vi "6812B_AC.vi"() -> ()   [LabVIEW 2019]
doc: "Shows how to generate a standard output."
uses:
  <instrlib>/Agilent 681x Series/Agilent 681x Series.lvlib
panel:
  out "PwrMeas":T1
  out "CurMeas":T2
  out "CUR":T3(graph)={"Peak Current"=0.0194168, "AC RMS Current"=0.00868389, "AC + DC RMS Current"=0.00868755}
  out "POT":T4(graph)={"Reactive Power"=0.130219, "Real Power"=0.000577786, "Apparent Power"=0.13022}
  in  "STOP":bool
  in  "Pulse Characteristic Value (%)":dbl=100.0 format="%#.4g"
  in  "Pulse Characteristic (0: Duty Cycle)":u16(ring) items=["Duty Cycle", "Pulse Width"]
  in  "Period (s)":dbl=10.0 format="%#.4g"
  in  "Trigger Delay (s)":dbl=10.0 format="%#.5g"
  in  "Pulse Count":dbl=1.0 format="%#.4g"
  in  "Voltage Mode (0: Fix)":u16(ring) items=["Fixed", "Step", "Pulse", "List"]
  in  "Triggered Voltage Amplitude (V)":dbl=1.0 format="%#.4g"
  in  "Peak Current Limit (13 A)":dbl=13.0 format="%#.4g"
  in  "RMS Current Limit (1 A)":dbl=1.0 format="%#.4g"
  in  "Voltage Amplitude (1.0 V)":dbl=1.0 format="%#.4g"
  in  "Output Frequency (60 Hz)":dbl=60.0 format="%#.4g"
  in  "Output Waveform Type (0: Sinusoid)":u16(ring) items=["Sinusoid", "Square", "Clipped Sinusoid", "User Specified"]
  in  "VISA resource name":refnum<visa-resource-name>
  # "(c) 2008-2021 National Instruments Corp.  ALL RIGHTS RESERVED."
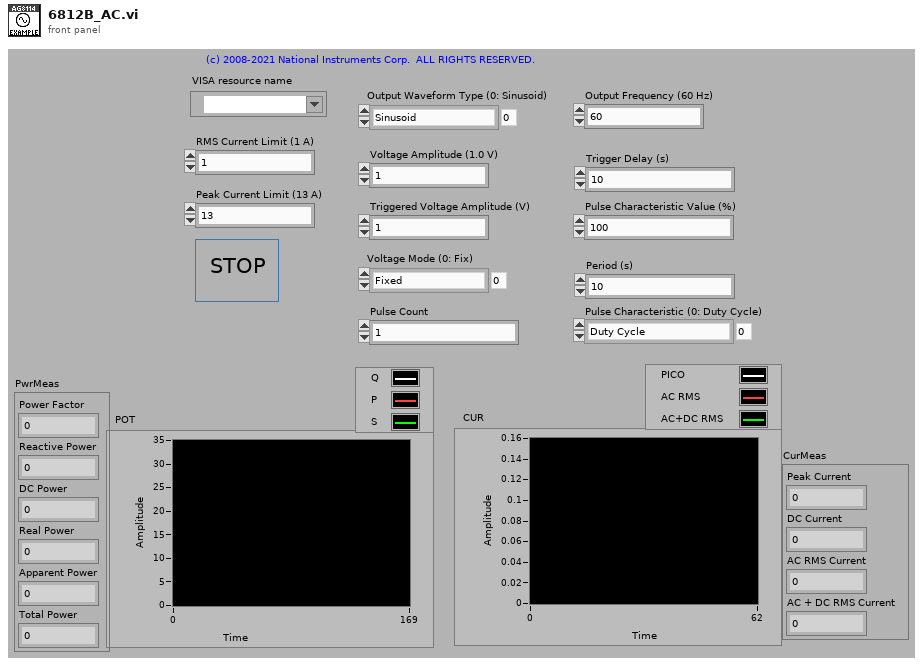
[diagram p1: front panel]
types:
  T1 = cluster{"Power Factor":dbl, "Reactive Power":dbl, "DC Power":dbl, "Real Power":dbl, "Apparent Power":dbl, "Total Power":dbl}
  T2 = cluster{"Peak Current":dbl, "DC Current":dbl, "AC RMS Current":dbl, "AC + DC RMS Current":dbl}
  T3 = cluster{"Peak Current":dbl, "AC RMS Current":dbl, "AC + DC RMS Current":dbl}
  T4 = cluster{"Reactive Power":dbl, "Real Power":dbl, "Apparent Power":dbl}
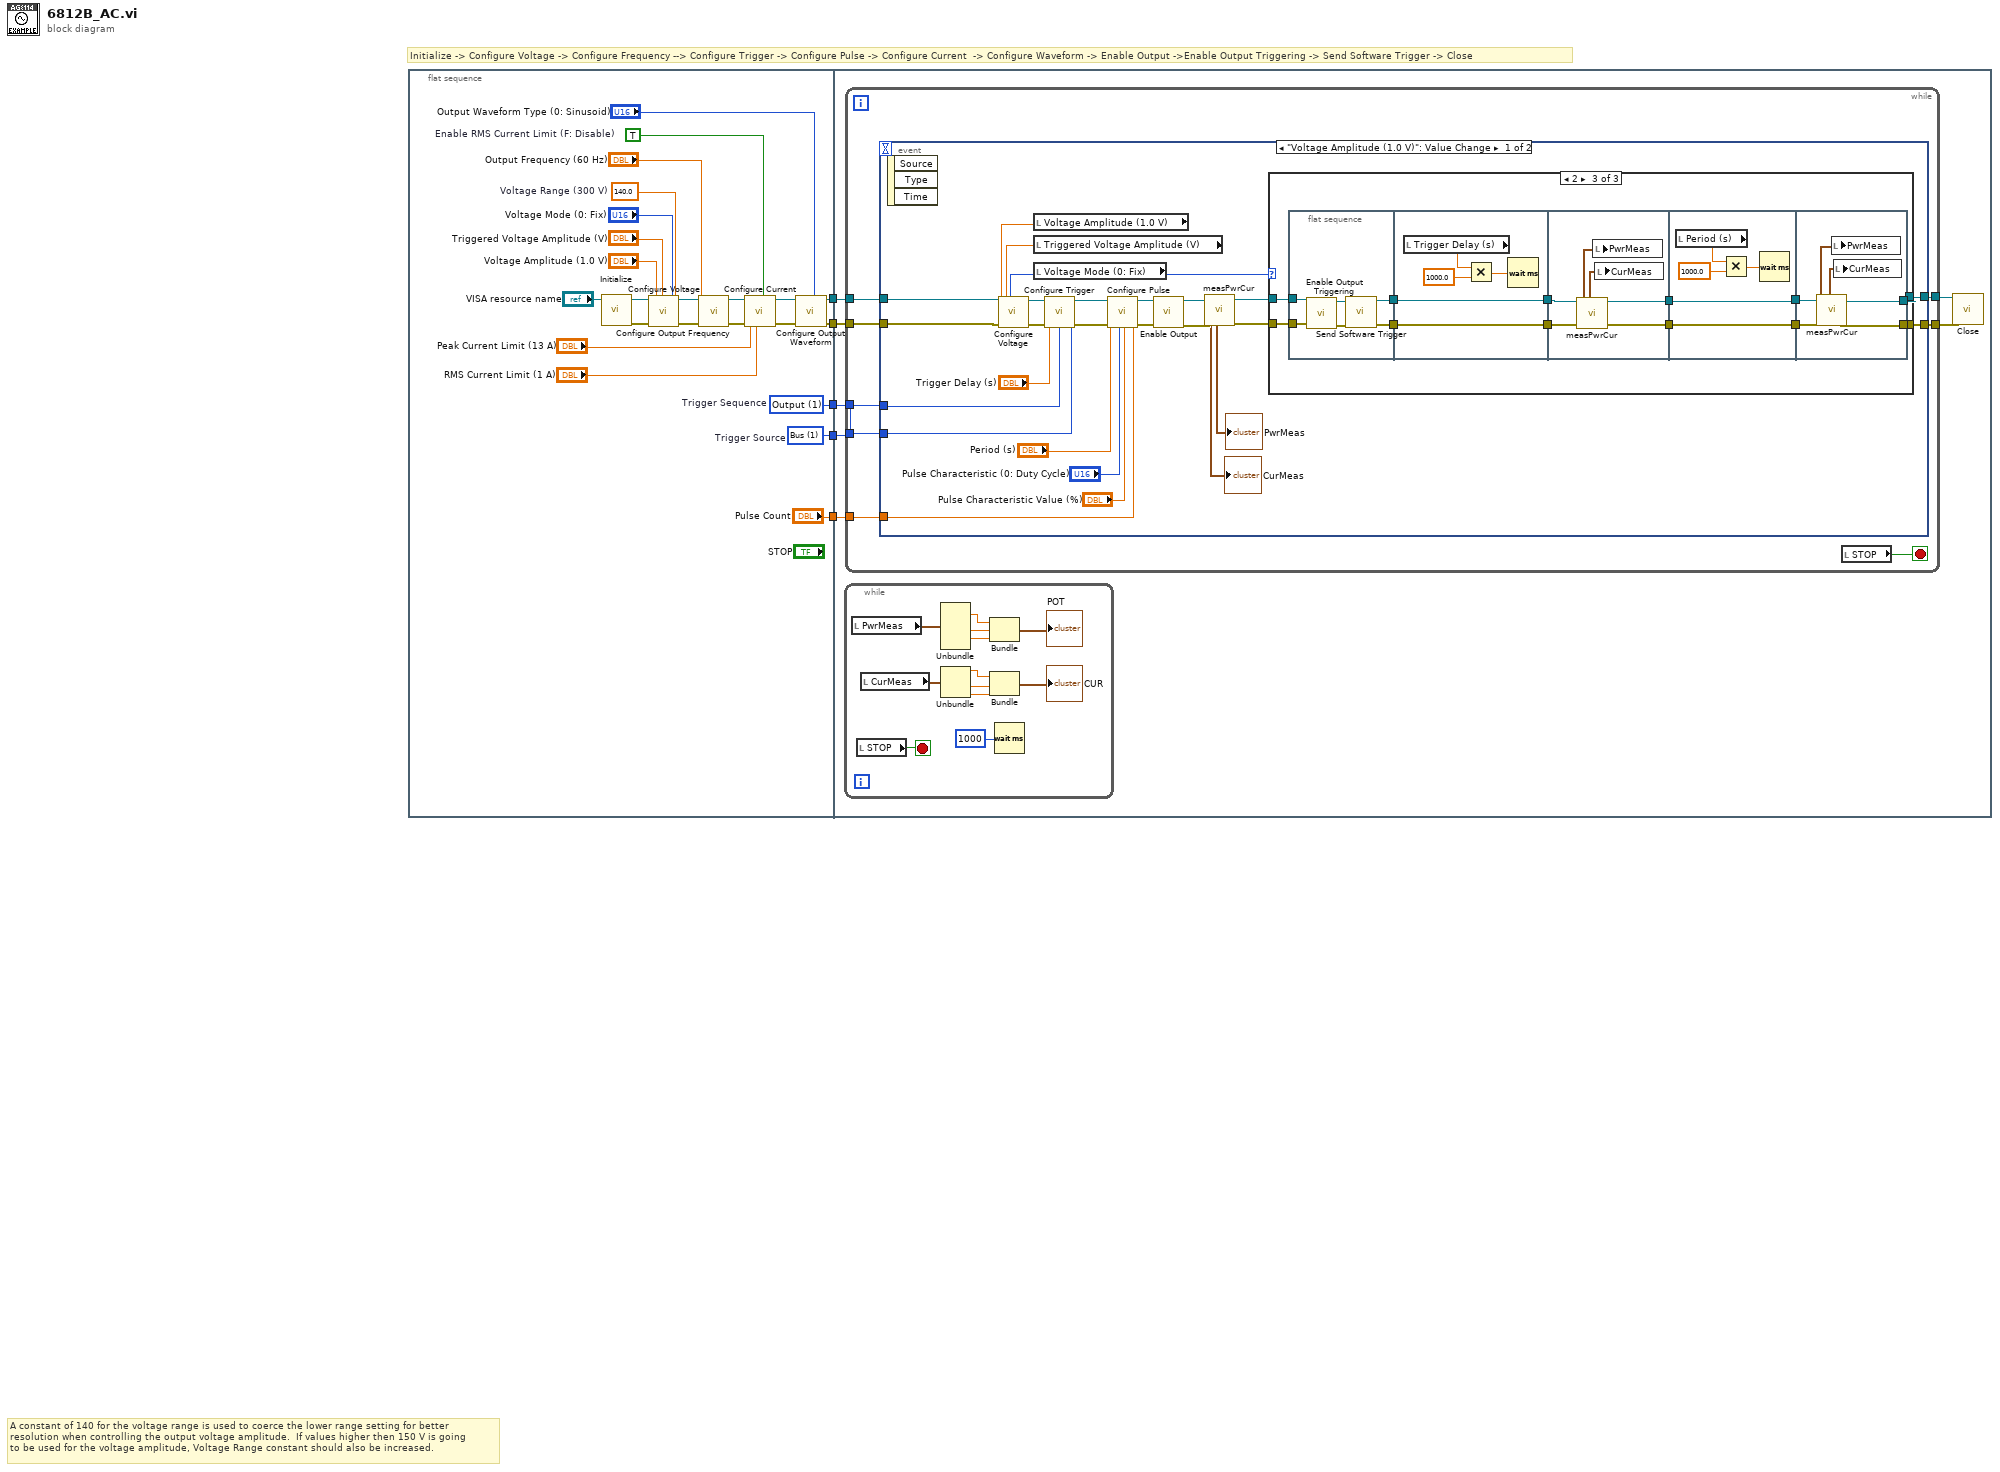
[diagram p0: block diagram]
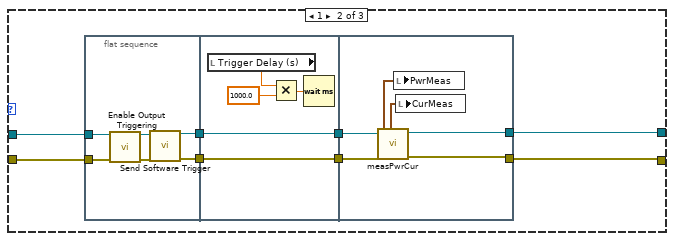
[diagram p3: hidden frame]
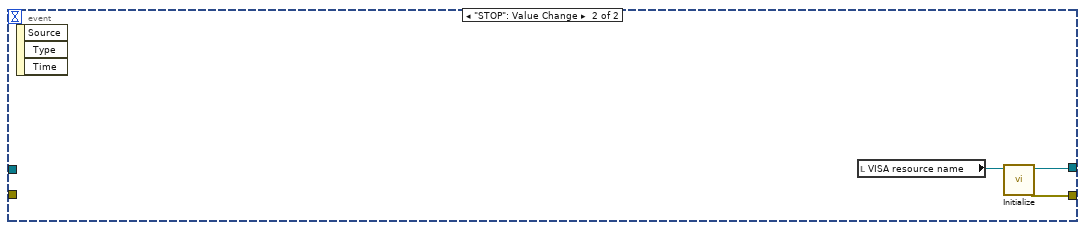
[diagram p4: hidden frame]
diagram:
  # "Initialize -> Configure Voltage -> Configure Frequency --> Configure Trigger -> Configure Pulse -> Configure Current  -> Configure Waveform -> Enable Output ->Enable Output Triggering -> Send Software Trigger -> Close"
  # "A constant of 140 for the voltage range is used to coerce the lower range setting for better\nresolution when controlling the output voltage amplitude.  If values higher then 150 V is going\nto be used for the voltage amplitude, Voltage Range constant should also be increased."
  n1 = flat-sequence {
    tunnel: [w13] -> w5
    tunnel: [w12] -> w4
    tunnel: [w8] -> w3
    tunnel: [w7] -> w2
    tunnel: ["Pulse Count"] -> w1
    tunnel: w5 -> [w34]
    tunnel: w4 -> [w33]
    tunnel: w3 -> [w29]
    tunnel: w2 -> [w30]
    tunnel: w1 -> [w28]
    frame #0 {
      w8 = 1 items=["Immediate", "Bus", "External", "Phase", "Trigger Out"]  # Trigger Source
      w7 = 1 items=["Output"=1, "Synchronous Source"=2, "Measurement"=3]  # Trigger Sequence
      w20 = TRUE  # Enable RMS Current Limit (F: Disable)
      w9 = 140.0  # Voltage Range (300 V)
      n2 = call <instrlib>:"Initialize.vi"("VISA resource name"="VISA resource name") -> ("error out"=w15:errorcluster)  [unwired: 9 in, 1 out]
      n3 = call <instrlib>:"Configure Voltage.vi"("VISA resource name"="VISA resource name", "Triggered Voltage Amplitude (1.0 V)"="Triggered Voltage Amplitude (V)", "Voltage Range (300 V)"=w9, "Voltage Amplitude (1.0 V)"="Voltage Amplitude (1.0 V)", "Voltage Mode (0: Fix)"="Voltage Mode (0: Fix)", "error in (no error)"=w15) -> ("VISA resource name out"=w24:refnum<visa-resource-name>, "error out"=w25:errorcluster)  [unwired: 8 in]
      n4 = call <instrlib>:"Configure Output Frequency.vi"("VISA resource name"=w24, "Output Frequency (60 Hz)"="Output Frequency (60 Hz)", "error in (no error)"=w25) -> ("VISA resource name out"=w11:refnum<visa-resource-name>, "error out"=w10:errorcluster)  [unwired: 11 in]
      n5 = call <instrlib>:"Configure Current.vi"("VISA resource name"=w11, "Enable RMS Current Limit (F: Disable)"=w20, "RMS Current Limit (1 A)"="RMS Current Limit (1 A)", "error in (no error)"=w10, "Peak Current Limit (13 A)"="Peak Current Limit (13 A)") -> ("VISA resource name out"=w26:refnum<visa-resource-name>, "error out"=w27:errorcluster)  [unwired: 9 in]
      n6 = call <instrlib>:"Configure Output Waveform.vi"("VISA resource name"=w26, "Output Waveform Type (0: Sinusoid)"="Output Waveform Type (0: Sinusoid)", "error in (no error)"=w27) -> ("VISA resource name out"=w13:refnum<visa-resource-name>, "error out"=w12:errorcluster)  [unwired: 11 in]
    }
    frame #1 {
      n7 = while {
        stop <- w150 stop-if-true
        n8 = local read "PwrMeas"() -> (w148:T1)
        n9 = local read "STOP"() -> (w150:bool)
        n10 = local read "CurMeas"() -> (w143:T2)
        n11 = Unbundle(w148) -> ("Reactive Power"=w145:dbl, "Real Power"=w147:dbl, "Apparent Power"=w146:dbl)  [unwired: 3 out]
        n12 = Unbundle(w143) -> ("Peak Current"=w142:dbl, "AC RMS Current"=w141:dbl, "AC + DC RMS Current"=w140:dbl)  [unwired: 1 out]
        n13 = Bundle("Reactive Power"=w145, "Real Power"=w147, "Apparent Power"=w146) -> (→"POT":T4)  [unwired: 1 in]
        n14 = Bundle("Peak Current"=w142, "AC RMS Current"=w141, "AC + DC RMS Current"=w140) -> (→"CUR":T3)  [unwired: 1 in]
        n15 = Wait (ms)(milliseconds to wait=u32 1000) -> ()  [unwired: 1 out]
      }
      n16 = while {
        tunnel: w34 -> [w42]
        tunnel: w33 -> [w41]
        tunnel: [w35] -> w32
        tunnel: [w36] -> w31
        tunnel: w30 -> [w39]
        tunnel: w29 -> [w38]
        tunnel: w28 -> [w37]
        stop <- w40 stop-if-true
        n17 = event shown="[0] \"Voltage Amplitude (1.0 V)\": Value Change" {
          selector: _ -> [_ _]
          dyn-events: _ -> [_ _]
          timeout: _ -> [_ _]
          tunnel: w42 -> [w66 _]
          tunnel: w41 -> [w65 _]
          tunnel: w39 -> [w55 _]
          tunnel: w38 -> [w54 _]
          tunnel: w37 -> [w49 _]
          tunnel: [w47 w136] -> w36
          tunnel: [w46 w137] -> w35
          event "Voltage Amplitude (1.0 V)": Value Change {
            n18 = event-data() -> ()  [unwired: 1 in, 3 out]
            n19 = local read "Voltage Amplitude (1.0 V)"() -> (w64:dbl)
            n20 = local read "Triggered Voltage Amplitude (V)"() -> (w48:dbl)
            n21 = local read "Voltage Mode (0: Fix)"() -> (w45:u16)
            n22 = call <instrlib>:"Configure Voltage.vi"("VISA resource name"=w66, "Triggered Voltage Amplitude (1.0 V)"=w48, "Voltage Amplitude (1.0 V)"=w64, "Voltage Mode (0: Fix)"=w45, "error in (no error)"=w65) -> ("VISA resource name out"=w61:refnum<visa-resource-name>, "error out"=w60:errorcluster)  [unwired: 9 in]
            n23 = call <instrlib>:"Configure Trigger.vi"("VISA resource name"=w61, "Trigger Sequence (1: Output 1)"=w55, "Trigger Source (0: Immediate)"=w54, "error in (no error)"=w60, "Trigger Delay (0 s)"="Trigger Delay (s)") -> ("VISA resource name out"=w62:refnum<visa-resource-name>, "error out"=w63:errorcluster)  [unwired: 9 in]
            n24 = call <instrlib>:"Configure Pulse.vi"("VISA resource name"=w62, "Pulse Count (1)"=w49, "Period (0.0333 s)"="Period (s)", "error in (no error)"=w63, "Pulse Characteristic (0: Duty Cycle)"="Pulse Characteristic (0: Duty Cycle)", "Pulse Characteristic Value (50)"="Pulse Characteristic Value (%)") -> ("VISA resource name out"=w59:refnum<visa-resource-name>, "error out"=w58:errorcluster)  [unwired: 8 in]
            n25 = call <instrlib>:"Enable Output.vi"("VISA resource name"=w59, "error in (no error)"=w58) -> ("VISA resource name out"=w68:refnum<visa-resource-name>, "error out"=w67:errorcluster)  [unwired: 12 in]
            n26 = call "measPwrCur.vi"("VISA resource name"=w68, "error in (no error)"=w67) -> ("PwrMeas"=→"PwrMeas":T1, "CurMeas"=→"CurMeas":T2, "VISA resource name out"=w57:refnum<visa-resource-name>, "error out"=w56:errorcluster)  [unwired: 3 in]
            n27 = case shown="2" w45 {
              tunnel: w57 -> [w70 w78 w101]
              tunnel: w56 -> [w69 w77 w100]
              tunnel: [w69 w72 w96] -> w47
              tunnel: [w70 w71 w97] -> w46
              frame 0, Default {
              }
              frame 1 {
                n28 = flat-sequence {
                  tunnel: w78 -> [w82]
                  tunnel: w77 -> [w81]
                  tunnel: [w80] -> w75
                  tunnel: [w79] -> w73
                  tunnel: [w89] -> w76
                  tunnel: w75 -> [w89]
                  tunnel: [w88] -> w74
                  tunnel: w73 -> [w88]
                  tunnel: w76 -> [w93]
                  tunnel: w74 -> [w90]
                  tunnel: [w91] -> w72
                  tunnel: [w92] -> w71
                  frame #0 {
                    n29 = call <instrlib>:"Enable Output Triggering.vi"("VISA resource name"=w82, "error in (no error)"=w81) -> ("VISA resource name out"=w83:refnum<visa-resource-name>, "error out"=w84:errorcluster)  [unwired: 12 in]
                    n30 = call <instrlib>:"Send Software Trigger.vi"("VISA resource name"=w83, "error in (no error)"=w84) -> ("VISA resource name out"=w80:refnum<visa-resource-name>, "error out"=w79:errorcluster)  [unwired: 12 in]
                  }
                  frame #1 {
                    n31 = local read "Trigger Delay (s)"() -> (w87:dbl)
                    n32 = Multiply(x=w87, y=1000.0) -> (x*y=w85:dbl)
                    n33 = Wait (ms)(milliseconds to wait=w85) -> ()  [unwired: 1 out]
                  }
                  frame #2 {
                    n34 = call "measPwrCur.vi"("VISA resource name"=w93, "error in (no error)"=w90) -> ("PwrMeas"=w94:T1, "CurMeas"=w95:T2, "VISA resource name out"=w92:refnum<visa-resource-name>, "error out"=w91:errorcluster)  [unwired: 3 in]
                    n35 = local write "PwrMeas"(w94) -> ()
                    n36 = local write "CurMeas"(w95) -> ()
                  }
                }
              }
              frame 2 {
                n37 = flat-sequence {
                  tunnel: [w111] -> w107
                  tunnel: [w110] -> w106
                  tunnel: w101 -> [w109]
                  tunnel: w100 -> [w108]
                  tunnel: [w118] -> w105
                  tunnel: w107 -> [w118]
                  tunnel: [w117] -> w104
                  tunnel: w106 -> [w117]
                  tunnel: w105 -> [w124]
                  tunnel: w104 -> [w123]
                  tunnel: [w122] -> w103
                  tunnel: [w121] -> w102
                  tunnel: w103 -> [w125]
                  tunnel: w102 -> [w126]
                  tunnel: [w126] -> w99
                  tunnel: [w125] -> w98
                  tunnel: w99 -> [w134]
                  tunnel: w98 -> [w133]
                  tunnel: [w132] -> w97
                  tunnel: [w131] -> w96
                  frame #0 {
                    n38 = call <instrlib>:"Enable Output Triggering.vi"("VISA resource name"=w109, "error in (no error)"=w108) -> ("VISA resource name out"=w112:refnum<visa-resource-name>, "error out"=w113:errorcluster)  [unwired: 12 in]
                    n39 = call <instrlib>:"Send Software Trigger.vi"("VISA resource name"=w112, "error in (no error)"=w113) -> ("VISA resource name out"=w111:refnum<visa-resource-name>, "error out"=w110:errorcluster)  [unwired: 12 in]
                  }
                  frame #1 {
                    n40 = local read "Trigger Delay (s)"() -> (w116:dbl)
                    n41 = Multiply(x=w116, y=1000.0) -> (x*y=w114:dbl)
                    n42 = Wait (ms)(milliseconds to wait=w114) -> ()  [unwired: 1 out]
                  }
                  frame #2 {
                    n43 = call "measPwrCur.vi"("VISA resource name"=w124, "error in (no error)"=w123) -> ("PwrMeas"=w119:T1, "CurMeas"=w120:T2, "VISA resource name out"=w121:refnum<visa-resource-name>, "error out"=w122:errorcluster)  [unwired: 3 in]
                    n44 = local write "PwrMeas"(w119) -> ()
                    n45 = local write "CurMeas"(w120) -> ()
                  }
                  frame #3 {
                    n46 = local read "Period (s)"() -> (w127:dbl)
                    n47 = Multiply(x=w127, y=1000.0) -> (x*y=w129:dbl)
                    n48 = Wait (ms)(milliseconds to wait=w129) -> ()  [unwired: 1 out]
                  }
                  frame #4 {
                    n49 = call "measPwrCur.vi"("VISA resource name"=w134, "error in (no error)"=w133) -> ("PwrMeas"=w135:T1, "CurMeas"=w130:T2, "VISA resource name out"=w132:refnum<visa-resource-name>, "error out"=w131:errorcluster)  [unwired: 3 in]
                    n50 = local write "PwrMeas"(w135) -> ()
                    n51 = local write "CurMeas"(w130) -> ()
                  }
                }
              }
            }
          }
          event "STOP": Value Change {
            n52 = event-data() -> ()  [unwired: 1 in, 3 out]
            n53 = local read "VISA resource name"() -> (w138:refnum<visa-resource-name>)
            n54 = call <instrlib>:"Initialize.vi"("VISA resource name"=w138) -> ("error out"=w136:errorcluster, "VISA resource name out"=w137:refnum<visa-resource-name>)  [unwired: 9 in]
          }
        }
        n55 = local read "STOP"() -> (w40:bool)
      }
      n56 = call <instrlib>:"Close.vi"("error in (no error)"=w31, "VISA resource name"=w32) -> ()  [unwired: 9 in, 1 out]
    }
  }
